vi "dfd_Validate Quantization Wls (Adv).vi"(5 "Coef b/v quantizer":T1={"source"=0, "wl"=16, "iwl"=1, "overflow mode"=enum."Wrap", "rounding mode"=enum."Truncation", "signed?"=TRUE} {"source" items=["Coefficients a/k"=0, "Coefficients b/v"=7, "Input"=1, "Output"=2, "Multiplicand"=3, "Product"=4, "Sum"=5, "Delay"=6]}, 6 "gain setting":cluster{"gain processing":u16, "gain wl":i16}={"gain processing"=0, "gain wl"=16} {"gain processing" items=["On Target", "On Host"]}, 7 "Coef a/k quantizer":T1={"source"=0, "wl"=16, "iwl"=1, "overflow mode"=enum."Wrap", "rounding mode"=enum."Truncation", "signed?"=TRUE} {"source" items=["Coefficients a/k"=0, "Coefficients b/v"=7, "Input"=1, "Output"=2, "Multiplicand"=3, "Product"=4, "Sum"=5, "Delay"=6]}, 8 "error in (no error)":errorcluster, 11 "filter in":T3={"mSRate_Fs"=1.0, "mSRate_Version"="1.0", "mSRate_Comments"="", "mSRate_OrgCoef"={"type"=enum."Undefined", "gain"=1.0, "coef a (k)"=[], "coef b (v)"=[]}, "mSRate_CurCoef"={"type"=enum."Undefined", "gain"=1.0, "coef a (k)"=[], "coef b (v)"=[]}, "mSRate_Quantized?"=FALSE, "mSRate_QCoef"={"type"=enum."Undefined", "gain"=1.0, "coef a (k)"=[], "coef b (v)"=[]}, "mSRate_QSettings"=[], "mSRate_Order"=0, "mSRate_Scaling"={"mSRate_ScaleByPowerOf2?"=FALSE, "mSRate_ScaleType"=enum."No Norm"}} {"mSRate_QSettings"."source" items=["Coef a/k"=0, "Coef b/v"=7, "Input"=1, "Output"=2, "Multiplicand"=3, "Product"=4, "Sum"=5, "Delay"=6, "Gain"=8]}) -> (0 "error out":errorcluster, 3 "filter out":T3={"mSRate_Fs"=1.0, "mSRate_Version"="1.0", "mSRate_Comments"="", "mSRate_OrgCoef"={"type"=enum."Undefined", "gain"=1.0, "coef a (k)"=[], "coef b (v)"=[]}, "mSRate_CurCoef"={"type"=enum."Undefined", "gain"=1.0, "coef a (k)"=[], "coef b (v)"=[]}, "mSRate_Quantized?"=FALSE, "mSRate_QCoef"={"type"=enum."Undefined", "gain"=1.0, "coef a (k)"=[], "coef b (v)"=[]}, "mSRate_QSettings"=[], "mSRate_Order"=0, "mSRate_Scaling"={"mSRate_ScaleByPowerOf2?"=FALSE, "mSRate_ScaleType"=enum."No Norm"}} {"mSRate_QSettings"."source" items=["Coef a/k"=0, "Coef b/v"=7, "Input"=1, "Output"=2, "Multiplicand"=3, "Product"=4, "Sum"=5, "Delay"=6, "Gain"=8]})   [LabVIEW 2017, in "NI_DigFilter_FXP.lvlib"]
uses:
  <vilib>/addons/Digital Filter Design/NI_DigFilter_FXP.lvlib
  <vilib>/addons/Digital Filter Design/_Objects.llb/DFD Filter Obj.ctl
  <vilib>/addons/Digital Filter Design/_Objects.llb/DFD Filter Coef.ctl
  <vilib>/addons/Digital Filter Design/_Objects.llb/DFD Filter Structure Type Selector.ctl
  <vilib>/addons/Digital Filter Design/_Objects.llb/dfd_Internal Quantization Settings.ctl
  <vilib>/addons/Digital Filter Design/_Objects.llb/dfd_Internal Quantization Srcs.ctl
  <vilib>/addons/Digital Filter Design/_Objects.llb/DFD Coef Norm Type.ctl
  <vilib>/addons/Digital Filter Design/_Objects.llb/DFD Quantization Settings.ctl
  <vilib>/addons/Digital Filter Design/_Objects.llb/DFD Quantization Sources.ctl
  <vilib>/addons/Digital Filter Design/NI_DigFilterLicensed.lvlib
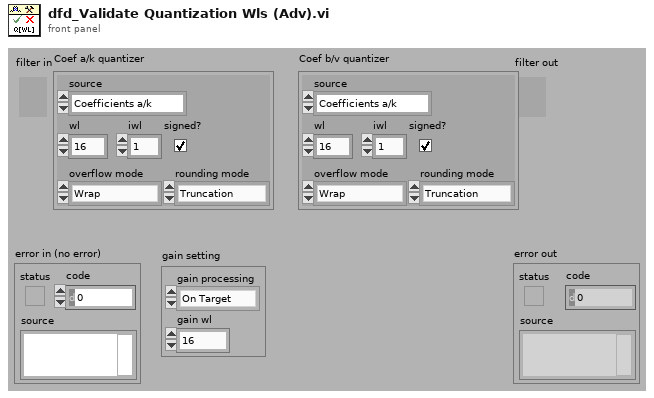
[diagram p1: front panel]
types:
  T1 = typedef "NI_DigFilterLicensed.lvlib/DFD Quantization Settings.ctl" = cluster{"source":T2, "wl":i16, "iwl":i16, "overflow mode":enum16{"Saturation", "Wrap"}, "rounding mode":enum16{"Nearest", "Truncation"}, "signed?":bool}
  T2 = typedef "NI_DigFilterLicensed.lvlib/DFD Quantization Sources.ctl" = u16
  T3 = typedef "NI_DigFilterLicensed.lvlib/DFD Filter Obj.ctl" = cluster{"mSRate_Fs":dbl, "mSRate_Version":string, "mSRate_Comments":string, "mSRate_OrgCoef":T4, "mSRate_CurCoef":T4, "mSRate_Quantized?":bool, "mSRate_QCoef":T4, "mSRate_QSettings":T6[], "mSRate_Order":i32, "mSRate_Scaling":cluster{"mSRate_ScaleByPowerOf2?":bool, "mSRate_ScaleType":T8}}
  T4 = typedef "NI_DigFilterLicensed.lvlib/DFD Filter Coef.ctl" = cluster{"type":T5, "gain":dbl, "coef a (k)":dbl[], "coef b (v)":dbl[]}
  T5 = typedef "NI_DigFilterLicensed.lvlib/DFD Filter Structure Type Selector.ctl" = enum16{"Undefined", "FIR Direct Form", "FIR Direct Form Transposed", "FIR Symmetric", "FIR Antisymmetric", "IIR Direct Form I", "IIR Direct Form I Transposed", "IIR Direct Form II", "IIR Direct Form II Transposed", "IIR Cascaded Second Order Sections Form I", "IIR Cascaded Second Order Sections Form I Transposed", "IIR Cascaded Second Order Sections Form II", "IIR Cascaded Second Order Sections Form II Transposed", "Lattice Allpass (basic sections)", "Lattice Allpass (one multiplier sections)", "Lattice Allpass (normalized sections)", "Lattice AR (basic sections)", "Lattice AR (one multiplier sections)", "Lattice AR (normalized sections)", "Lattice MA (minimum phase)", "Lattice MA (maximum phase)", "Lattice ARMA (basic sections)", "Lattice ARMA (one multiplier sections)", "Lattice ARMA (normalized sections)"}
  T6 = typedef "NI_DigFilterLicensed.lvlib/dfd_Internal Quantization Settings.ctl" = cluster{"source":T7, "wl":i16, "iwl":i16, "overflow mode":enum16{"Saturation", "Wrap"}, "rounding mode":enum16{"Nearest", "Truncation"}, "signed?":bool}
  T7 = typedef "NI_DigFilterLicensed.lvlib/dfd_Internal Quantization Srcs.ctl" = u16
  T8 = typedef "NI_DigFilterLicensed.lvlib/DFD Coef Norm Type.ctl" = enum16{"No Norm", "Time Domain 1-Norm", "Time Domain 2-Norm", "Time Domain Inf-Norm"}
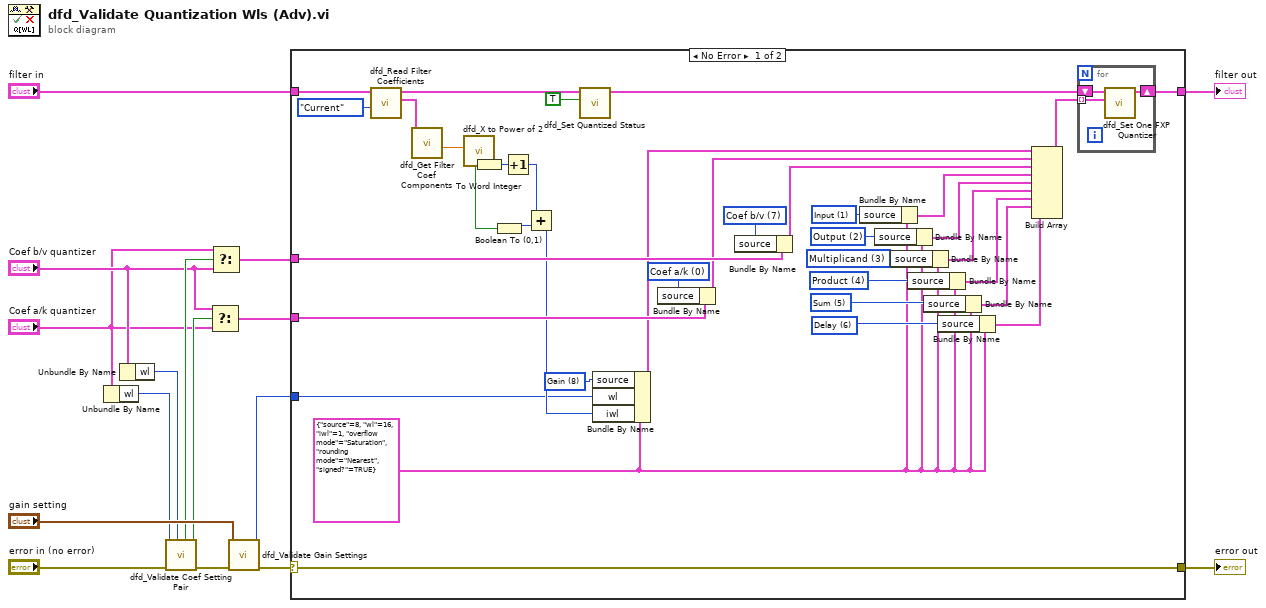
[diagram p0: block diagram]
diagram:
  n1 = Unbundle By Name("Coef a/k quantizer") -> ("wl"=w3:i16)
  n2 = Unbundle By Name("Coef b/v quantizer") -> ("wl"=w4:i16)
  n3 = call <vilib>:"dfd_Validate Coef Setting Pair.vi"("coef b/v wl"=w4, "error in (no error)"="error in (no error)", "coef a/k wl"=w3) -> ("error out"=w11:errorcluster, "a/k selector"=w6:bool, "b/v selector"=w5:bool)  [unwired: 6 out]
  n4 = Select(t="Coef b/v quantizer", s=w6, f="Coef a/k quantizer") -> (s? t:f=w13:T1)
  n5 = Select(t="Coef a/k quantizer", s=w5, f="Coef b/v quantizer") -> (s? t:f=w12:T1)
  n6 = call <vilib>:"dfd_Validate Gain Settings.vi"("error in (no error)"=w11, "gain setting"="gain setting") -> ("error out"=w9:errorcluster, "gain wl"=w7:i16)  [unwired: 8 out]
  n7 = case shown="No Error" w9 {
    selector: w9 -> [w43 w59]
    tunnel: [w43 w59] -> w16
    tunnel: "filter in" -> [w54 w58]
    tunnel: [w22 w58] -> w14
    tunnel: w7 -> [w36 _]
    tunnel: w13 -> [w42 _]
    tunnel: w12 -> [w40 _]
    frame No Error {
      w17 = T6 {"source"=8, "wl"=16, "iwl"=1, "overflow mode"=enum."Saturation", "rounding mode"=enum."Nearest", "signed?"=TRUE} ("quantizer")
      w30 = T7 6 items=["Coef a/k"=0, "Coef b/v"=7, "Input"=1, "Output"=2, "Multiplicand"=3, "Product"=4, "Sum"=5, "Delay"=6, "Gain"=8] ("source")
      w31 = T7 5 items=["Coef a/k"=0, "Coef b/v"=7, "Input"=1, "Output"=2, "Multiplicand"=3, "Product"=4, "Sum"=5, "Delay"=6, "Gain"=8] ("source")
      w32 = T7 4 items=["Coef a/k"=0, "Coef b/v"=7, "Input"=1, "Output"=2, "Multiplicand"=3, "Product"=4, "Sum"=5, "Delay"=6, "Gain"=8] ("source")
      w33 = T7 3 items=["Coef a/k"=0, "Coef b/v"=7, "Input"=1, "Output"=2, "Multiplicand"=3, "Product"=4, "Sum"=5, "Delay"=6, "Gain"=8] ("source")
      w34 = T7 2 items=["Coef a/k"=0, "Coef b/v"=7, "Input"=1, "Output"=2, "Multiplicand"=3, "Product"=4, "Sum"=5, "Delay"=6, "Gain"=8] ("source")
      w35 = T7 1 items=["Coef a/k"=0, "Coef b/v"=7, "Input"=1, "Output"=2, "Multiplicand"=3, "Product"=4, "Sum"=5, "Delay"=6, "Gain"=8] ("source")
      w45 = T7 7 items=["Coef a/k"=0, "Coef b/v"=7, "Input"=1, "Output"=2, "Multiplicand"=3, "Product"=4, "Sum"=5, "Delay"=6, "Gain"=8] ("source")
      w41 = T7 0 items=["Coef a/k"=0, "Coef b/v"=7, "Input"=1, "Output"=2, "Multiplicand"=3, "Product"=4, "Sum"=5, "Delay"=6, "Gain"=8] ("source")
      w49 = T7 8 items=["Coef a/k"=0, "Coef b/v"=7, "Input"=1, "Output"=2, "Multiplicand"=3, "Product"=4, "Sum"=5, "Delay"=6, "Gain"=8] ("source")
      n8 = call <vilib>:"dfd_Read Filter Coefficients.vi"("coef source"=enum16{"Original", "Current", "Quantized"}."Current", "filter in"=w54) -> ("filter coef"=w52:T4, "filter out"=w47:T3)  [unwired: 1 in, 7 out]
      n9 = call <vilib>:"dfd_Get Filter Coef Components.vi"("filter coef"=w52) -> ("gain"=w51:dbl)  [unwired: 1 in, 9 out]
      n10 = call <vilib>:"dfd_X to Power of 2.vi"("x"=w51) -> ("n"=w50:dbl, "is 2^n?"=w37:bool)  [unwired: 9 out]
      n11 = To Word Integer(number=w50) -> (16bit integer=w48:i16)
      n12 = Boolean To (0,1)(Boolean=w37) -> (0, 1=w38:i16)
      n13 = Increment(x=w48) -> (x+1=w44:i16)
      n14 = Add(x=w44, y=w38) -> (x+y=w39:i16)
      n15 = call <vilib>:"dfd_Set Quantized Status.vi"("quantized?"=TRUE, "filter in"=w47) -> ("filter out"=w23:T3)  [unwired: 1 in, 8 out]
      n16 = Bundle By Name(cluster=w17, "source"=w49, "wl"=w36, "iwl"=w39) -> (w21:T6)
      n17 = Bundle By Name(cluster=w42, "source"=w41) -> (w20:T1)
      n18 = Bundle By Name(cluster=w40, "source"=w45) -> (w19:T1)
      n19 = Bundle By Name(cluster=w17, "source"=w35) -> (w18:T6)
      n20 = Bundle By Name(cluster=w17, "source"=w34) -> (w24:T6)
      n21 = Bundle By Name(cluster=w17, "source"=w33) -> (w29:T6)
      n22 = Bundle By Name(cluster=w17, "source"=w32) -> (w28:T6)
      n23 = Bundle By Name(cluster=w17, "source"=w31) -> (w27:T6)
      n24 = Bundle By Name(cluster=w17, "source"=w30) -> (w26:T6)
      n25 = Build Array(w21, w20, w19, w18, w24, w29, w28, w27, w26) -> (w25:T6[])
      n26 = for {
        tunnel: w25 -> [w57] mode=indexing
        shift-right: [w55] -> w22
        shift-left: w23 -> [w56]
        n27 = call <vilib>:"dfd_Set One FXP Quantizer.vi"("quantization settings"=w57, "filter in"=w56) -> ("filter out"=w55:T3)  [unwired: 1 in, 8 out]
      }
    }
    frame Error {
    }
  }
  "filter out" <- w14
  "error out" <- w16
